vi "Parse Location.vi"(11 "Location":string) -> (3 "Query Parameters":variant)   [LabVIEW 2013]
uses:
  <vilib>/LabVIEW Open Source Project/OpenURI/uri/URI.lvclass/URI.ctl
  <vilib>/LabVIEW Open Source Project/OpenURI/components/query/URI-Component.Query.lvclass/URI-Component.Query.ctl
  <vilib>/LabVIEW Open Source Project/OpenURI/components/query/Get Key-Value Pairs.vi
  <vilib>/LabVIEW Open Source Project/OpenURI/uri/URI.lvclass
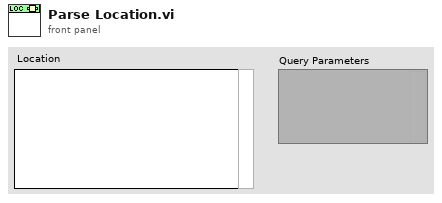
[diagram p1: front panel]
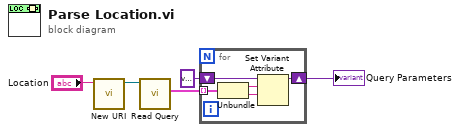
[diagram p0: block diagram]
diagram:
  n1 = call <vilib>:"New URI.vi"("URI"="Location") -> ("URI"=w5:refnum<class "URI.lvclass">)  [unwired: 9 in, 1 out]
  n2 = call <vilib>:"Read Query.vi"("URI in"=w5) -> ("Query"=w4:cluster{"argument":string, "value":string}[])  [unwired: 8 in, 2 out]
  n3 = for {
    tunnel: w4 -> [w10] mode=indexing
    shift-right: [w7] -> w1
    shift-left: variant -> [w6]
    n4 = Unbundle(w10) -> ("argument"=w9:string, "value"=w8:string)
    n5 = Set Variant Attribute(Variant=w6, name=w9, value=w8) -> (Variant out=w7:variant)  [unwired: 1 in, 2 out]
  }
  "Query Parameters" <- w1
